vi "Move.vi"(6 "Absolute (0.0 um)":dbl format="%.1f", 7 "Direction (1: Down)":enum16{"Up", "Down", "Absolute"}(ring)=enum."Down", 8 "error in (no error)":errorcluster {"code" format="%.0x"}, 9 "Step (0.0 um)":dbl format="%.1f", 10 "Device Number (1)":i32=1, 11 "VISA Resource Name":refnum<visa-resource-name>) -> (0 "error out":errorcluster {"code" format="%.0x"}, 2 "Result":string, 3 "VISA Resource Name Out":refnum<visa-resource-name>)   [LabVIEW 2020]
uses:
  Drivers/Olympus IX BX Series/Olympus IX BX Series.lvlib
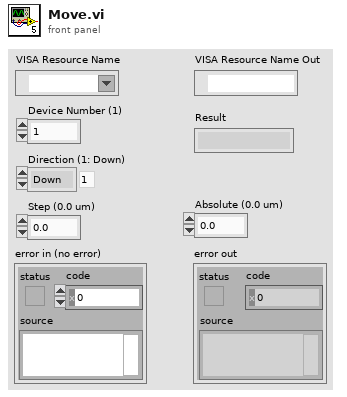
[diagram p1: front panel]
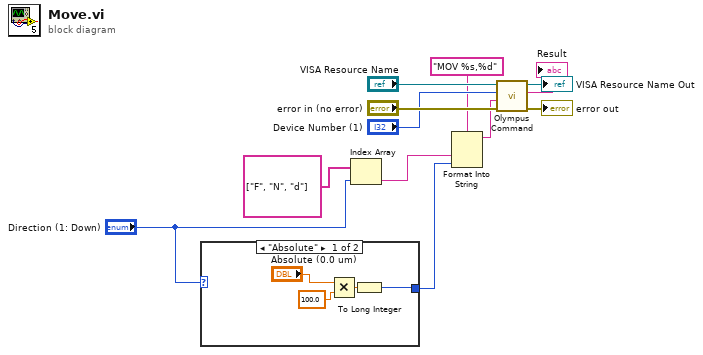
[diagram p0: block diagram]
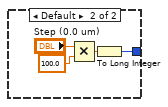
[diagram p2: hidden frame]
diagram:
  n1 = case shown="\"Absolute\"" "Direction (1: Down)" {
    tunnel: [w13 w17] -> w10
    frame "Absolute" {
      n2 = Multiply(x="Absolute (0.0 um)", y=100.0) -> (x*y=w15:dbl)
      n3 = To Long Integer(number=w15) -> (32bit integer=w13:i32)
    }
    frame Default {
      n4 = Multiply(x="Step (0.0 um)", y=100.0) -> (x*y=w18:dbl)
      n5 = To Long Integer(number=w18) -> (32bit integer=w17:i32)
    }
  }
  n6 = Index Array(array=string[] ["F", "N", "d"], index="Direction (1: Down)") -> (element=w11:string)
  n7 = Format Into String(format string="MOV %s,%d", w11, w10) -> (resulting string=w5:string)  [unwired: 2 in, 1 out]
  n8 = call "Olympus Command.vi"("error in (no error)"="error in (no error)", "Command string"=w5, "Device Number (1)"="Device Number (1)", "VISA Resource Name"="VISA Resource Name") -> ("error out"=→"error out":errorcluster, "Result"=→"Result":string, "VISA Resource Name Out"=→"VISA Resource Name Out":refnum<visa-resource-name>)  [unwired: 5 in]
